vi "Item Picked Up.vi"(8 "error in (no error)":errorcluster, 10 "Item Picked Up":string, 11 "Customer in":refnum<class "Customer.lvclass">) -> (0 "error out":errorcluster, 3 "Customer out":refnum<class "Customer.lvclass">)   [LabVIEW 2020, in "Customer.lvclass"]
uses:
  Customer.lvclass
  Customer.lvclass/Customer.ctl
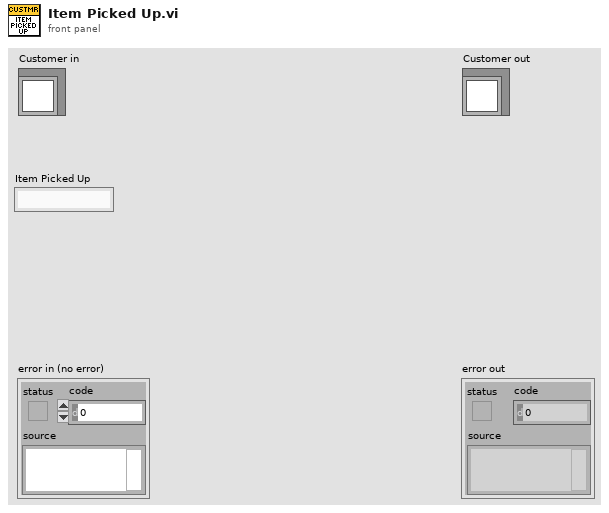
[diagram p1: front panel]
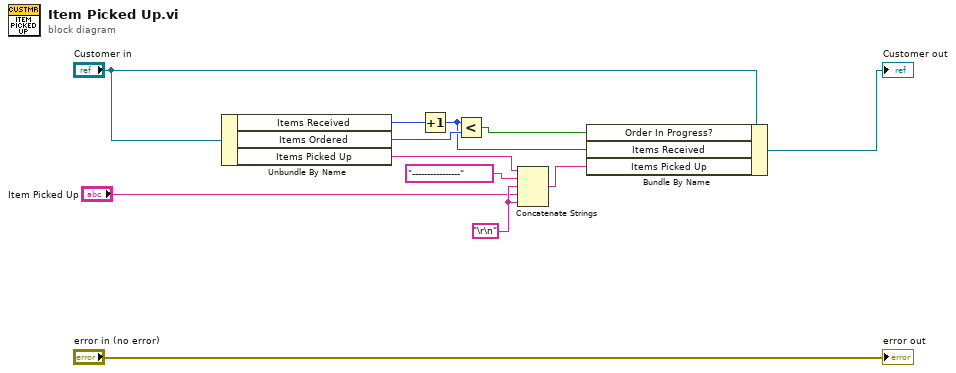
[diagram p0: block diagram]
diagram:
  w10 = "\r\n" ("End of Line Constant")
  n1 = Unbundle By Name("Customer in") -> ("Items Received"=w5:u32, "Items Ordered"=w4:u32, "Items Picked Up"=w8:string)
  n2 = Increment(x=w5) -> (x+1=w2:u32)
  n3 = Less?(x=w2, y=w4) -> (x < y?=w3:bool)
  n4 = Concatenate Strings(w8, "----------------" ("string"), w10, "Item Picked Up", w10) -> (w6:string)
  n5 = Bundle By Name(cluster="Customer in", "Order In Progress?"=w3, "Items Received"=w2, "Items Picked Up"=w6) -> (→"Customer out":refnum<class "Customer.lvclass">)
  "error out" <- "error in (no error)"
